vi "Cached Read Boolean.vi"(8 "error in (no error)":errorcluster, 10 "CVT_Boolean in":refnum<class "CVT_Boolean.lvclass">, 11 "Current Value Table in":refnum<class "Current Value Table.lvclass">) -> (0 "error out":errorcluster, 2 "value":bool, 3 "Current Value Table out":refnum<class "Current Value Table.lvclass">)   [LabVIEW 2024, in "Current Value Table.lvlib" / "Current Value Table.lvclass"]
uses:
  Current Value Table.lvclass
  Current Value Table.lvclass/Current Value Table.ctl
  CVT_Boolean/CVT_Boolean.lvclass
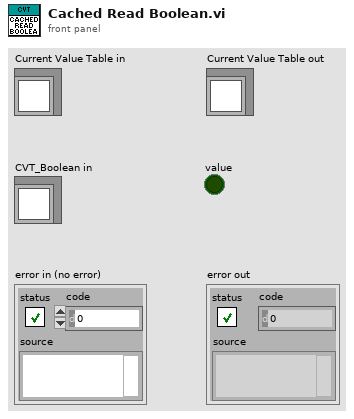
[diagram p1: front panel]
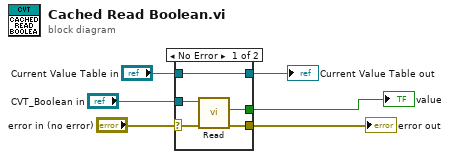
[diagram p0: block diagram]
diagram:
  n1 = case shown="No Error" "error in (no error)" {
    selector: "error in (no error)" -> [w8 w13]
    tunnel: [w7 w13] -> w5
    tunnel: [w11 w12] -> w3
    tunnel: "Current Value Table in" -> [w11 w12]
    tunnel: "CVT_Boolean in" -> [w10 _]
    tunnel: [w9 _] -> w1
    frame No Error {
      n2 = call-dynamic "Read.vi"("error in (no error)"=w8, "CVT_Boolean in"=w10) -> ("error out"=w7:errorcluster, "value"=w9:bool)  [unwired: 7 in, 1 out]
    }
    frame Error {
    }
  }
  "error out" <- w5
  "Current Value Table out" <- w3
  "value" <- w1
